vi "VI Tree.vi"   [LabVIEW 2021, in "Thread.lvlib"]
uses:
  Thread.lvlib
  fbdaca25-0451-4e1e-a589-3362d264cc44.vi
  Cache Action.ctl
types:
  T1 = typedef "Thread.lvlib/Cache Action.ctl" = enum8{"noop", "get", "add", "remove", "remove_by_ref"}
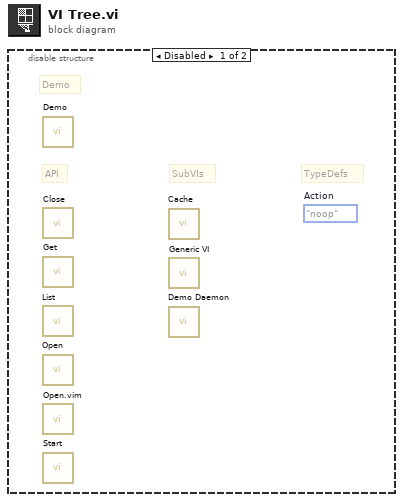
[diagram p0: block diagram]
diagram:
  n1 = disable-structure shown="Disabled" {
    frame Disabled {
      (unwired) Cache_Action."noop"  # Action
      # "Demo"
      # "TypeDefs"
      # "SubVIs"
      # "API"
      n2 = call "Demo.vi"() -> ()  [unwired: 12 in]
      n3 = call "Close.vi"() -> ()  [unwired: 11 in, 1 out]
      n4 = call "Get.vi"() -> ()  [unwired: 8 in, 4 out]
      n5 = call "List.vi"() -> ()  [unwired: 10 in, 2 out]
      n6 = call "Open.vi"() -> ()  [unwired: 9 in, 3 out]
      n7 = call "Open.vim"() -> ()  [unwired: 9 in, 3 out]
      n8 = call "Start.vi"() -> ()  [unwired: 9 in, 3 out]
      n9 = call "Cache.vi"() -> ()  [unwired: 7 in, 5 out]
      n10 = call "Generic VI.vi"() -> ()  [unwired: 9 in, 3 out]
      n11 = call "Demo Daemon.vi"() -> ()  [unwired: 12 in]
    }
    frame Enabled {
    }
  }
